vi "main.vi"() -> ()   [LabVIEW 2013]
uses:
  <vilib>/addons/internet/telnet/telnet.llb/Telnet Session.ctl
  <vilib>/Platform/TimedLoop/XDataNode/timing_clust.ctl
  <vilib>/Platform/TimedLoop/XDataNode/nitl_modes.ctl
  <vilib>/Platform/TimedLoop/XDataNode/wakeup.ctl
  FGV/STANDARD/Action.ctl
  <vilib>/Utility/config.llb/Read Key (Path).vi
  <vilib>/Utility/config.llb/Write Key (Path).vi
  <vilib>/Instr/_visa.llb/VISA Configure Serial Port (Instr).vi
  <vilib>/Platform/TimedLoop/XDataNode/XDataNode.xnode
  <vilib>/Platform/TimedLoop/XDataNode/XDNodeRunTimeDep.lvlib
  <vilib>/Utility/config.llb/NI_LVConfig.lvlib
panel:
  out "SettingsFile":path=path "D:/JD/PROJETS/wrk/WORKING_DIR"
  out "Tftp":T1={"HostIP"="192.168.1.200", "HostPort"=23, "ClientIP"="192.168.1.200"}
  out "Telnet":cluster{"HostIP":string, "HostPort":u16}={"HostIP"="192.168.1.200", "HostPort"=23}
  out "Error Out":errorcluster caption="Sortie d'erreur"
  in  "Serial_Port":refnum<visa-resource-name> caption="Serial Port"
  out "Serial_Connected":bool caption="Serial"
  in  "Serial_Connect":bool caption="Cmd_Tx"
  in  "Serial_Clear":bool
  in  "Serial_Console":string caption="Console"
  out "telnet connection":T2
  in  "BTN_Quit":bool
  in  "LauncherRef":refnum<vi>
  in  "entrée d'erreur":errorcluster caption="sortie d'erreur"
  out "sortie d'erreur":errorcluster
  in  "ONGLETS":enum32{"CONFIGURATION", "LOW_LEVEL", "COMMANDS"}(tab)
  in  "Host_IpAddress":string="192.168.1.200" caption="GHB Address"
  in  "MyIpList":string(combo) caption="My IP address"
  in  "WorkingDir":path=path "D:/JD/PROJETS/wrk/WORKING_DIR"
  in  "Host_TelnetPort":u16=23 caption="Telnet Port"
  in  "Host_TftpPort":u16=69 caption="Tftp Port"
  in  "OpenWorkingDir":bool
  in  "Telnet_Connect":bool
  in  "Telnet_Tx":bool caption="Cmd_Tx"
  in  "Telnet_Cmd":string caption="Cmd"
  in  "Telnet_Console":string caption="Console"
  in  "Telnet_Clear":bool
  out "Telnet_Connected":bool caption="Telnet"
  in  "Tftp_RemotePath":string
  out "Tftp_Status":bool caption="Status"
  in  "Tftp_LocalPath":path=path "D:/JD/PROJETS/wrk/TESTS"
  in  "Tftp_Get":bool
  in  "Tftp_Put":bool
  out "Tftp_Connected":bool caption="Tftp"
  in  "Cmd_ReservoirSet":bool caption="Cmd_Tx"
  in  "Cmd_ReservoirGet":bool caption="Cmd_Tx"
  in  "Cmd_Arroser":bool caption="Cmd_Tx"
  in  "Cmd_GetState":bool caption="Cmd_Tx"
  in  "Cmd_PutFile":bool caption="Cmd_Tx"
  in  "Cmd_GetFile":bool caption="Cmd_Tx"
  in  "FileList":i32(listbox)
  in  "Cmd_Reboot":bool caption="Cmd_Tx"
  in  "Cmd_ListFiles":bool caption="Cmd_Tx"
  in  "Cmd_Rename":bool caption="Cmd_Tx"
  in  "Cmd_Delete":bool caption="Cmd_Tx"
  in  "Cmd_Parameters":string caption="Parameters"
  in  "Cmd_Read":bool caption="Cmd_Tx"
  in  "Cmd_RtcGet":bool caption="Cmd_Tx"
  in  "Cmd_RtcSet":bool caption="Cmd_Tx"
  in  "Cmd_LogsGet":bool caption="Cmd_Tx"
  in  "Cmd_LogsClear":bool caption="Cmd_Tx"
  in  "Cmd_Console":string caption="Console"
  in  "Cmd_Clear":bool
  # "SERIAL"
  # "CONFIGURATION"
  # "TELNET"
  # "TFTP"
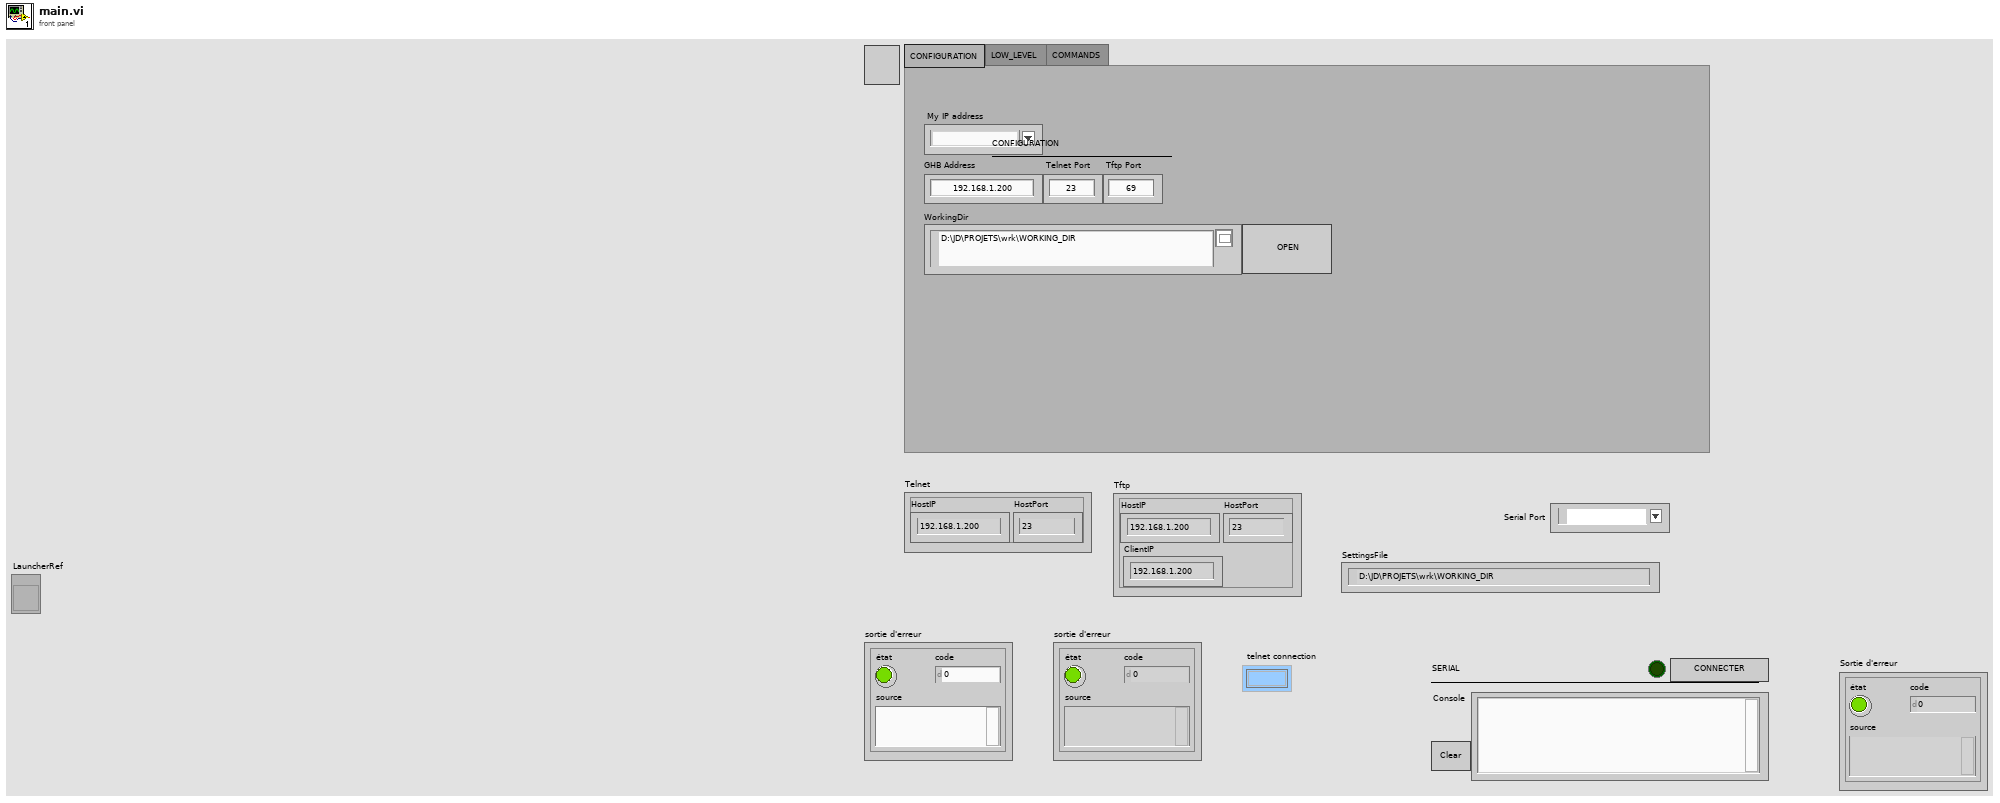
[diagram p1: front panel]
types:
  T1 = cluster{"HostIP":string, "HostPort":u16, "ClientIP":string}
  T2 = typedef "Telnet Session.ctl" = refnum<k1>
  T3 = enum32{"invalid app kind", "Development System", "Run Time System", "Student Edition", "Embedded LabVIEW", "Evaluation", "Custom"}
  T4 = typedef "Action.ctl" = enum16{"SET", "GET"}
  T5 = typedef "CtrlRef.ctl" = cluster{"Name":string, "Ref":refnum<vi>, "ClassName":string}
  T6 = typedef "NI_LVConfig.lvlib/Config Data RefNum.ctl" = refnum<k1>
  T7 = typedef "XDNodeRunTimeDep.lvlib/timing_clust.ctl" = cluster{"Expected End [f-1]":u64, "Actual End [f-1]":u64, "Finished Late? [f-1]":bool, "Expected End [i-1]":u64, "Actual End [i-1]":u64, "Finished Late? [i-1]":bool, "Expected Start [i]":u64, "Actual Start [i]":u64, "Expected Start [f]":u64, "Actual Start [f]":u64, "Source Name":string, "Structure Name":string, "Period":i64, "Deadline":i64, "Offset":i64, "Start":i64, "Priority":i32, "Timeout":i32, "Mode":T8, "Wakeup Reason":T9, "Error":errorcluster, "Source Type":string, "Secondary Source Type":string, "Global End Time":u64, "Global Start Time":u64, "Frame Duration":u64, "Iteration Duration":u64, "Assigned CPU":i32, "I/O Scan Engine Mode":u32}
  T8 = typedef "XDNodeRunTimeDep.lvlib/nitl_modes.ctl" = enum32{"No Change", "Process missed periods, maintain original phase", "Discard missed periods, maintain original phase", "Process missed periods, ignore original phase", "Discard missed periods, ignore original phase"}
  T9 = typedef "XDNodeRunTimeDep.lvlib/wakeup.ctl" = enum32{"Normal", "Aborted", "Asynchronous wakeup", "Timing source error", "Timed loop error", "Timeout"}
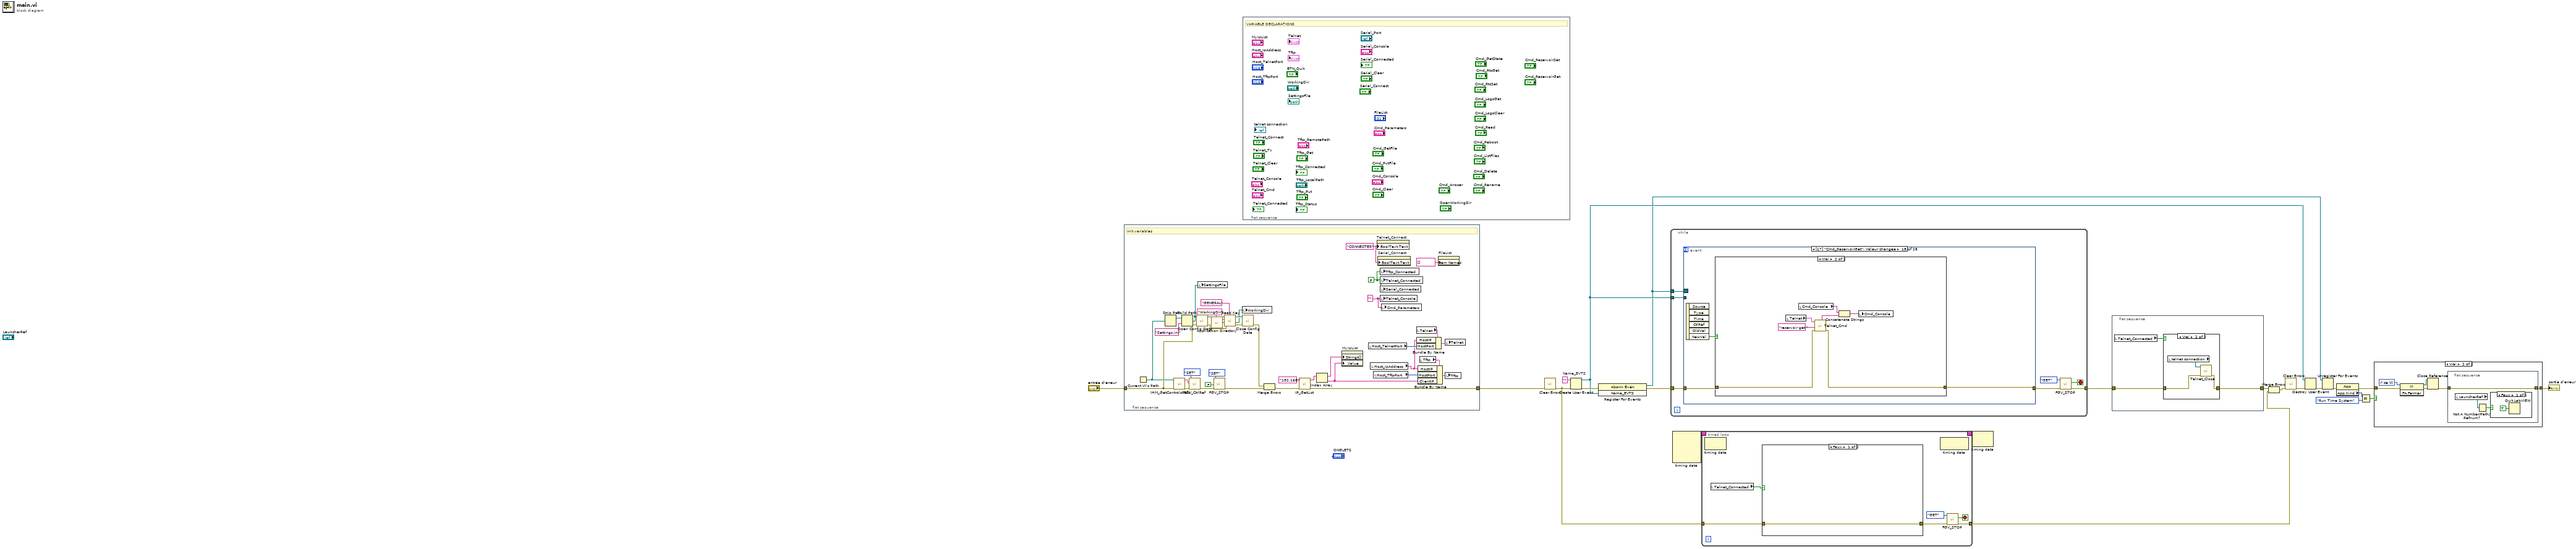
[diagram p0: block diagram]
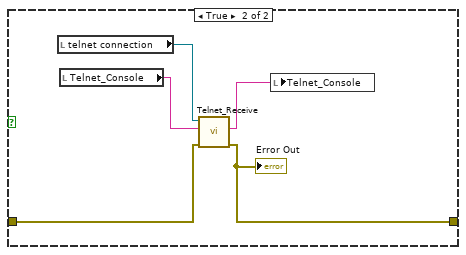
[diagram p3: hidden frame]
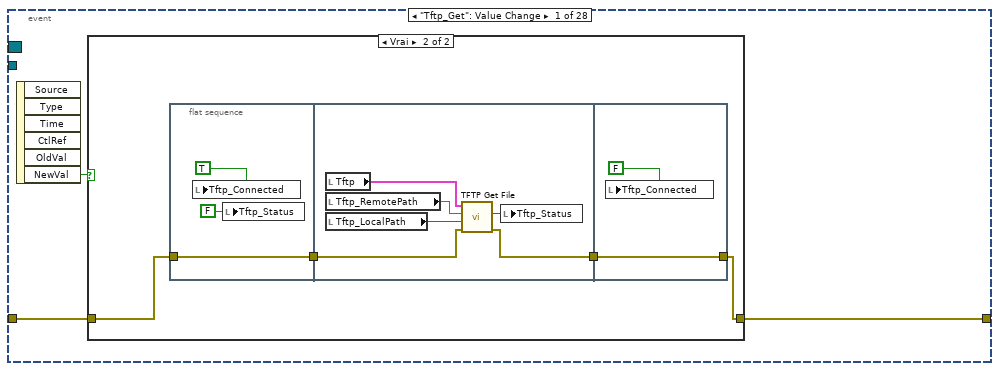
[diagram p6: hidden frame]
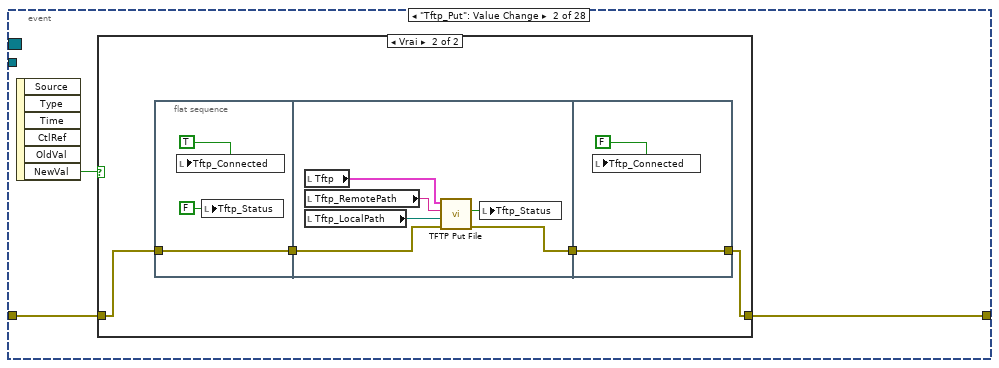
[diagram p8: hidden frame]
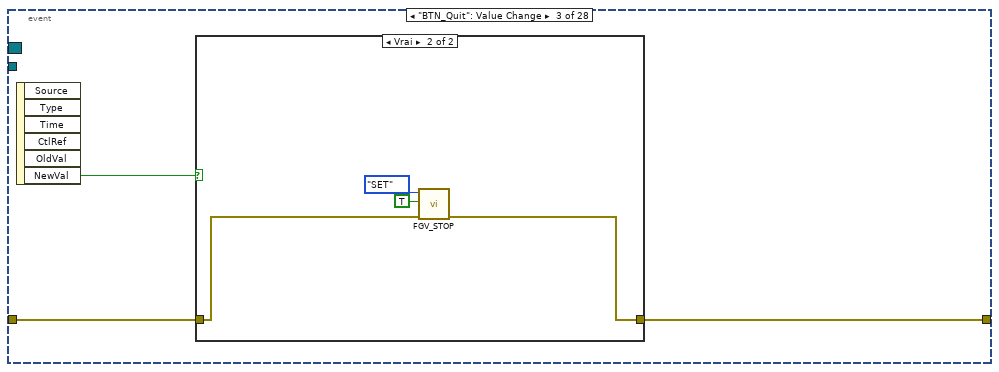
[diagram p10: hidden frame]
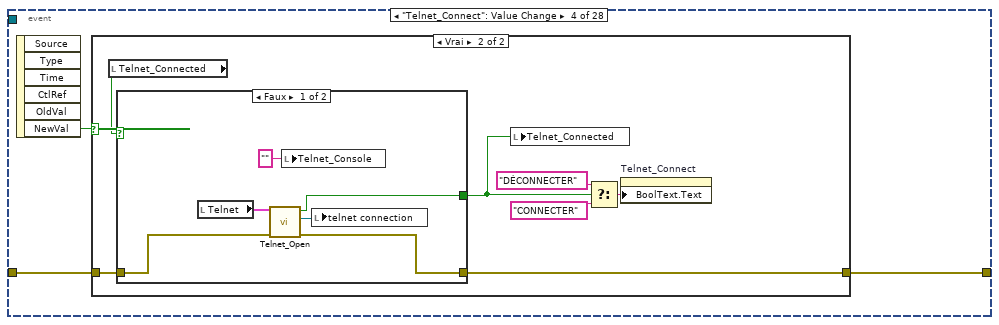
[diagram p12: hidden frame]
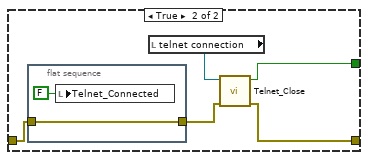
[diagram p14: hidden frame]
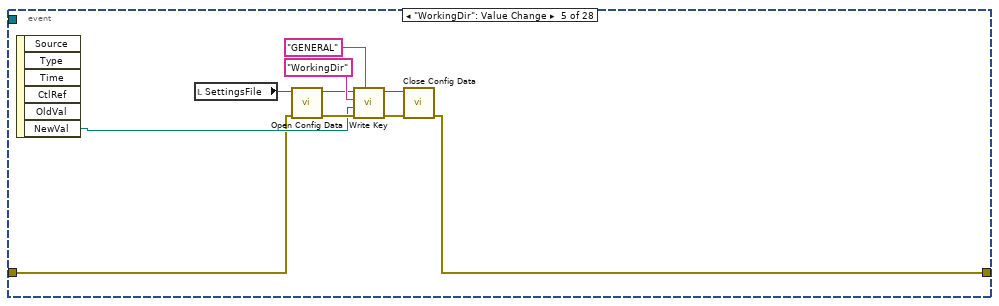
[diagram p15: hidden frame]
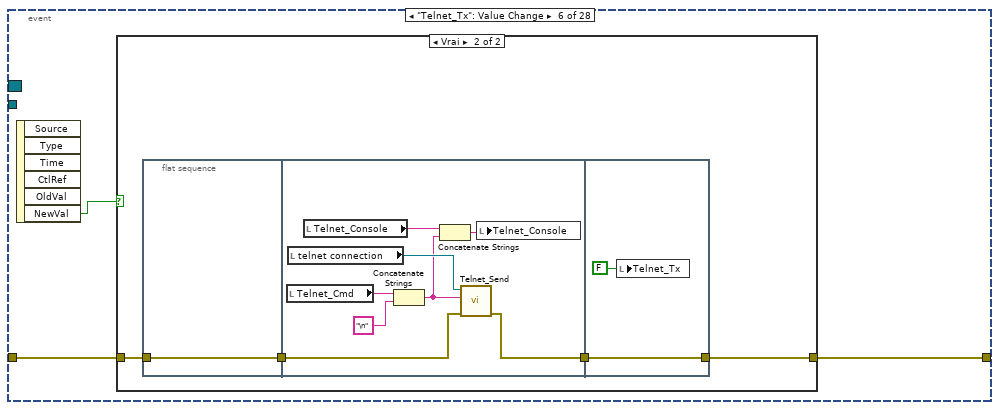
[diagram p16: hidden frame]
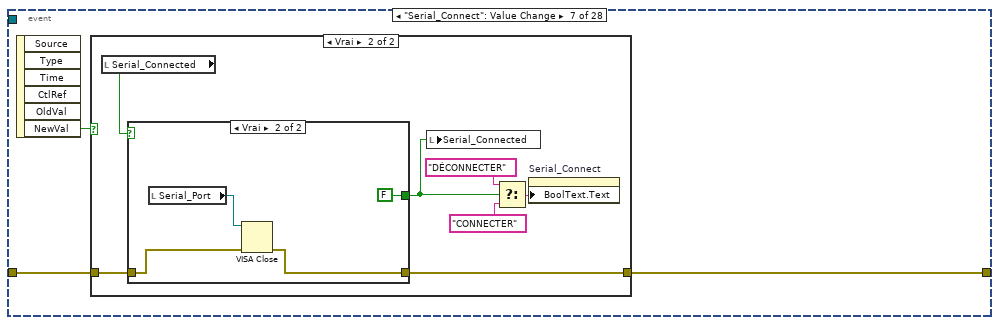
[diagram p18: hidden frame]
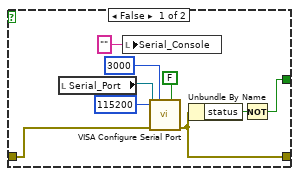
[diagram p20: hidden frame]
diagram:
  w22 = ""  # Name_EVTS
  n1 = flat-sequence {
    tunnel: [w51] -> w19
    tunnel: "entrée d'erreur" -> [w25]
    frame #0 {
      w54 = "" ("Telnet_Console")
      w56 = FALSE ("Telnet_Connected")
      w57 = "CONNECTER" ("Texte booléen.Texte")
      # "Init variables"
      n2 = Current VI's Path() -> (path=w37:path)
      n3 = Strip Path(path=w37) -> (stripped path=w38:path)  [unwired: 1 out]
      n4 = call "IHM_GetControlsRefs.vi"("Error In"=w25, "chemin du VI"=w37) -> ("Error Out"=w50:errorcluster, "CtrlsRefs_OUT"=w48:T5[])  [unwired: 8 in]
      n5 = Build Path(base path=w38, name or relative path="Settings.ini" ("nom ou chemin relatif")) -> (appended path=w24:path)
      n6 = call "FGV_CtrlRef.vi"("error in (no error)"=w50, "CtrlsRefs_IN"=w48, "Action"=Action."SET") -> ("error out"=w47:errorcluster)  [unwired: 7 in, 1 out]
      n7 = call <vilib>:"Open Config Data.vi"("error in (no error)"=w25, "configuration file path"=w24) -> ("error out"=w26:errorcluster, "refnum"=w35:T6)  [unwired: 7 in, 1 out]
      n8 = local write "SettingsFile"(w24) -> ()
      n9 = call <vilib>:"Application Directory.vi"() -> ("Application Directory"=w32:path)
      n10 = call "FGV_STOP.vi"("error in (no error)"=w47, "Data_IN"=FALSE, "Action"=Action."SET") -> ("error out"=w29:errorcluster)  [unwired: 7 in, 1 out]
      n11 = call-poly <vilib>:"Read Key.vi"("section"="GENERAL", "error in (no error)"=w26, "default value"=w32, "key"="WorkingDir", "refnum"=w35) -> ("error out"=w27:errorcluster, "value"=w31:path, "refnum out"=w34:T6)  [unwired: 3 in, 1 out]
      n12 = local write "WorkingDir"(w31) -> ()
      n13 = call <vilib>:"Close Config Data.vi"("error in (no error)"=w27, "refnum"=w34) -> ("error out"=w28:errorcluster)  [unwired: 8 in, 1 out]
      n14 = Merge Errors(w28, w29) -> (w30:errorcluster)
      n15 = call "IP_GetList.vi"("Error In"=w30, "MustContain"="192.168." ("expression régulière")) -> ("Error Out"=w51:errorcluster, "IP_List"=w52:string[])  [unwired: 8 in]
      n16 = Index Array(array=w52) -> (element=w42:string)  [unwired: 1 in]
      n17 = property on="MyIpList" class="ChneDér"("Strings[]"=w52, "Value"=w42) -> ()  [unwired: 2 in, 2 out]
      n18 = local read "Host_TelnetPort"() -> (w40:u16)
      n19 = local read "Host_IpAddress"() -> (w39:string)
      n20 = local read "Host_TftpPort"() -> (w41:u16)
      n21 = property on="Telnet_Connect" class="Bool (strict)"("BoolText.Text"=w57) -> ()  [unwired: 2 in, 2 out]
      n22 = property on="Serial_Connect" class="Bool (strict)"("BoolText.Text"=w57) -> ()  [unwired: 2 in, 2 out]
      n23 = local write "Tftp_Connected"(w56) -> ()
      n24 = local write "Telnet_Connected"(w56) -> ()
      n25 = local write "Serial_Connected"(w56) -> ()
      n26 = local write "Telnet_Console"(w54) -> ()
      n27 = local write "Cmd_Parameters"(w54) -> ()
      n28 = local read "Telnet"() -> (w43:cluster{"HostIP":string, "HostPort":u16})
      n29 = Bundle By Name(cluster=w43, "HostIP"=w39, "HostPort"=w40) -> (w44:cluster{"HostIP":string, "HostPort":u16})
      n30 = local read "Tftp"() -> (w46:T1)
      n31 = Bundle By Name(cluster=w46, "HostIP"=w39, "HostPort"=w41, "ClientIP"=w42) -> (w45:T1)
      n32 = property on="FileList" class="LstDér (strict)"("Item Names"=string[] [] ("Noms d'éléments")) -> ()  [unwired: 2 in, 2 out]
      n33 = local write "Tftp"(w45) -> ()
      n34 = local write "Telnet"(w44) -> ()
    }
  }
  n35 = flat-sequence {
    frame #0 {
      # "VARIABLE DECLARATIONS"
    }
  }
  n36 = call <vilib>:"Clear Errors.vi"("error in (no error)"=w19) -> ("error out"=w4:errorcluster)  [unwired: 6 in]
  n37 = Create User Event(user event datatype=w22, error in=w4) -> (user event=w9:refnum<user-event>, error out=w21:errorcluster)
  n38 = register-events(error in=w21, w9) -> (reference out=w8:refnum<event-registration>, error out=w7:errorcluster)  [unwired: 1 in]
  n39 = while {
    tunnel: w9 -> [w65]
    tunnel: w8 -> [w64]
    tunnel: [w62] -> w2
    tunnel: w7 -> [w60]
    stop <- w63 stop-if-true
    n40 = event shown="[17] \"Cmd_ReservoirGet\": Valeur changée" {
      selector: w64 -> [_ _ _ _ _ _ _ _ _ _ _ _ _ _ _ _ _ _ _ _ _ _ _ _ _ _ _ _]
      dyn-events: _ -> [_ _ _ _ _ _ _ _ _ _ _ _ _ _ _ _ _ _ _ _ _ _ _ _ _ _ _ _]
      timeout: _ -> [_ _ _ _ _ _ _ _ _ _ _ _ _ _ _ _ _ _ _ _ _ _ _ _ _ _ _ _]
      tunnel: w65 -> [_ _ _ _ _ _ _ _ _ _ _ _ _ _ _ _ _ _ _ _ _ _ _ _ _ _ _ _]
      tunnel: [w69 w87 w106 w115 w139 w149 w167 w192 w203 w214 w227 w239 w245 w248 w251 w254 w267 w280 w291 w304 w315 w329 w366 w372 w376 w380 w382 w394] -> w61
      tunnel: w60 -> [w68 w88 w105 w114 w140 w148 w168 w191 w204 w215 w228 w240 w245 w248 w251 w255 w268 w281 w292 w305 w316 w328 w366 w372 w376 w380 w383 w395]
      event "Tftp_Get": Value Change {
        n41 = event-data() -> ("NewVal"=w67:bool)  [unwired: 1 in, 5 out]
        n42 = case shown="Vrai" w67 {
          tunnel: [w70 w72] -> w69
          tunnel: w68 -> [w70 w73]
          frame False {
          }
          frame True {
            n43 = flat-sequence {
              tunnel: [w76] -> w74
              tunnel: w73 -> [w76]
              tunnel: w74 -> [w79]
              tunnel: [w78] -> w71
              tunnel: [w85] -> w72
              tunnel: w71 -> [w85]
              frame #0 {
                n44 = local write "Tftp_Connected"(TRUE ("Tftp_Connected")) -> ()
                n45 = local write "Tftp_Status"(FALSE ("TFTP_Status")) -> ()
              }
              frame #1 {
                n46 = local read "Tftp"() -> (w82:T1)
                n47 = local read "Tftp_RemotePath"() -> (w81:string)
                n48 = local read "Tftp_LocalPath"() -> (w80:path)
                n49 = call "TFTP Get File.vi"("error in (no error)"=w79, "local path"=w80, "remote path"=w81, "IpConf"=w82) -> ("error out"=w78:errorcluster, "Status"=w83:bool)  [unwired: 5 in, 1 out]
                n50 = local write "Tftp_Status"(w83) -> ()
              }
              frame #2 {
                n51 = local write "Tftp_Connected"(FALSE ("Tftp_Connected")) -> ()
              }
            }
          }
        }
      }
      event "Tftp_Put": Value Change {
        n52 = event-data() -> ("NewVal"=w86:bool)  [unwired: 1 in, 5 out]
        n53 = case shown="Vrai" w86 {
          tunnel: [w89 w91] -> w87
          tunnel: w88 -> [w89 w93]
          frame False {
          }
          frame True {
            n54 = flat-sequence {
              tunnel: w93 -> [w95]
              tunnel: [w95] -> w92
              tunnel: w92 -> [w98]
              tunnel: [w97] -> w90
              tunnel: [w104] -> w91
              tunnel: w90 -> [w104]
              frame #0 {
                n55 = local write "Tftp_Connected"(TRUE ("Tftp_Connected")) -> ()
                n56 = local write "Tftp_Status"(FALSE ("TFTP_Status")) -> ()
              }
              frame #1 {
                n57 = local read "Tftp"() -> (w101:T1)
                n58 = local read "Tftp_RemotePath"() -> (w100:string)
                n59 = local read "Tftp_LocalPath"() -> (w99:path)
                n60 = call "TFTP Put File.vi"("error in (no error)"=w98, "local path"=w99, "remote path"=w100, "IpConf"=w101) -> ("error out"=w97:errorcluster, "Status"=w102:bool)  [unwired: 5 in, 1 out]
                n61 = local write "Tftp_Status"(w102) -> ()
              }
              frame #2 {
                n62 = local write "Tftp_Connected"(FALSE ("Tftp_Connected")) -> ()
              }
            }
          }
        }
      }
      event "BTN_Quit": Value Change {
        n63 = event-data() -> ("NewVal"=w107:bool)  [unwired: 1 in, 5 out]
        n64 = case shown="Vrai" w107 {
          tunnel: [w108 w110] -> w106
          tunnel: w105 -> [w108 w111]
          frame False {
          }
          frame True {
            n65 = call "FGV_STOP.vi"("error in (no error)"=w111, "Data_IN"=TRUE, "Action"=Action."SET") -> ("error out"=w110:errorcluster)  [unwired: 7 in, 1 out]
          }
        }
      }
      event "Telnet_Connect": Value Change {
        n66 = event-data() -> ("NewVal"=w113:bool)  [unwired: 1 in, 5 out]
        n67 = case shown="Vrai" w113 {
          tunnel: [w116 w122] -> w115
          tunnel: w114 -> [w116 w123]
          frame False {
          }
          frame True {
            n68 = local read "Telnet_Connected"() -> (w121:bool)
            n69 = case shown="Faux" w121 {
              tunnel: w123 -> [w129 w130]
              tunnel: [w127 w134] -> w122
              tunnel: [w126 w132] -> w117
              frame False {
                n70 = local read "Telnet"() -> (w124:cluster{"HostIP":string, "HostPort":u16})
                n71 = call "Telnet_Open.vi"("Error In"=w129, "Telnet"=w124) -> ("Error Out"=w127:errorcluster, "telnet connection"=w128:T2, "Status"=w126:bool)  [unwired: 7 in]
                n72 = local write "Telnet_Console"("" ("Telnet_Console")) -> ()
                n73 = local write "telnet connection"(w128) -> ()
              }
              frame True {
                n74 = flat-sequence {
                  tunnel: [w136] -> w131
                  tunnel: w130 -> [w136]
                  frame #0 {
                    n75 = local write "Telnet_Connected"(FALSE ("Telnet_Connected")) -> ()
                  }
                }
                n76 = local read "telnet connection"() -> (w133:T2)
                n77 = call "Telnet_Close.vi"("Error In"=w131, "telnet connection"=w133) -> ("Error Out"=w134:errorcluster, "Connecté"=w132:bool)  [unwired: 8 in]
              }
            }
            n78 = local write "Telnet_Connected"(w117) -> ()
            n79 = Select(t="DÉCONNECTER" ("Texte booléen.Texte"), s=w117, f="CONNECTER" ("Texte booléen.Texte")) -> (s? t:f=w118:string)
            n80 = property on="Telnet_Connect" class="Bool (strict)"("BoolText.Text"=w118) -> ()  [unwired: 2 in, 2 out]
          }
        }
      }
      event "WorkingDir": Value Change {
        n81 = event-data() -> ("NewVal"=w141:path)  [unwired: 1 in, 5 out]
        n82 = local read "SettingsFile"() -> (w138:path)
        n83 = call <vilib>:"Open Config Data.vi"("error in (no error)"=w140, "configuration file path"=w138) -> ("error out"=w146:errorcluster, "refnum"=w142:T6)  [unwired: 7 in, 1 out]
        n84 = call-poly <vilib>:"Write Key.vi"("section"="GENERAL", "error in (no error)"=w146, "value"=w141, "key"="WorkingDir", "refnum"=w142) -> ("error out"=w145:errorcluster, "refnum out"=w143:T6)  [unwired: 4 in, 1 out]
        n85 = call <vilib>:"Close Config Data.vi"("error in (no error)"=w145, "refnum"=w143) -> ("error out"=w139:errorcluster)  [unwired: 8 in, 1 out]
      }
      event "Telnet_Tx": Value Change {
        n86 = event-data() -> ("NewVal"=w147:bool)  [unwired: 1 in, 5 out]
        n87 = case shown="Vrai" w147 {
          tunnel: [w150 w153] -> w149
          tunnel: w148 -> [w150 w154]
          frame False {
          }
          frame True {
            n88 = flat-sequence {
              tunnel: w154 -> [w155]
              tunnel: [w155] -> w152
              tunnel: w152 -> [w162]
              tunnel: [w161] -> w151
              tunnel: [w165] -> w153
              tunnel: w151 -> [w165]
              frame #0 {
              }
              frame #1 {
                n89 = local read "Telnet_Cmd"() -> (w158:string)
                n90 = local read "telnet connection"() -> (w163:T2)
                n91 = local read "Telnet_Console"() -> (w160:string)
                n92 = Concatenate Strings(w158, "\n") -> (w156:string)
                n93 = Concatenate Strings(w160, w156) -> (w159:string)
                n94 = call "Telnet_Send.vi"("Error In"=w162, "Data in"=w156, "telnet connection in"=w163) -> ("Error Out"=w161:errorcluster)  [unwired: 7 in, 1 out]
                n95 = local write "Telnet_Console"(w159) -> ()
              }
              frame #2 {
                n96 = local write "Telnet_Tx"(FALSE ("Telnet_Tx")) -> ()
              }
            }
          }
        }
      }
      event "Serial_Connect": Value Change {
        n97 = event-data() -> ("NewVal"=w166:bool)  [unwired: 1 in, 5 out]
        n98 = case shown="Vrai" w166 {
          tunnel: [w169 w175] -> w167
          tunnel: w168 -> [w169 w176]
          frame False {
          }
          frame True {
            n99 = local read "Serial_Connected"() -> (w171:bool)
            n100 = case shown="Vrai" w171 {
              tunnel: w176 -> [w182 w188]
              tunnel: [w179 w187] -> w175
              tunnel: [w177 FALSE] -> w172
              frame False {
                n101 = local read "Serial_Port"() -> (w183:refnum<visa-resource-name>)
                n102 = local write "Serial_Console"("" ("Telnet_Console")) -> ()
                n103 = call-poly "VISA Configure Serial Port"("VISA resource name"=w183, "timeout (10sec)"=u32 3000, "Enable Termination\nChar (T)"=FALSE ("Enable Termination\nChar (T)"), "baud rate (9600)"=u32 115200, "error in (no error)"=w182) -> ("error out"=w179:errorcluster)  [unwired: 9 in, 1 out]
                n104 = Unbundle By Name(w179) -> ("status"=w178:bool)
                n105 = Not(x=w178) -> (.not. x?=w177:bool)
              }
              frame True {
                n106 = local read "Serial_Port"() -> (w189:refnum<visa-resource-name>)
                n107 = VISA Close(VISA resource name=w189, error in (no error)=w188) -> (error out=w187:errorcluster)
              }
            }
            n108 = local write "Serial_Connected"(w172) -> ()
            n109 = Select(t="DÉCONNECTER" ("Texte booléen.Texte"), s=w172, f="CONNECTER" ("Texte booléen.Texte")) -> (s? t:f=w170:string)
            n110 = property on="Serial_Connect" class="Bool (strict)"("BoolText.Text"=w170) -> ()  [unwired: 2 in, 2 out]
          }
        }
      }
      event "Cmd_ListFiles": Value Change {
        n111 = event-data() -> ("NewVal"=w190:bool)  [unwired: 1 in, 5 out]
        n112 = case shown="Vrai" w190 {
          tunnel: [w193 w198] -> w192
          tunnel: w191 -> [w193 w200]
          frame False {
          }
          frame True {
            n113 = local read "Telnet"() -> (w201:cluster{"HostIP":string, "HostPort":u16})
            n114 = local read "Cmd_Console"() -> (w196:string)
            n115 = call "Telnet_Cmd.vi"("Error In"=w200, "Cmd"="ls", "Host"=w201) -> ("Error Out"=w198:errorcluster, "DataLines"=w197:string[], "Console"=w194:string)  [unwired: 5 in, 1 out]
            n116 = property on="FileList" class="LstDér (strict)"("Item Names"=w197) -> ()  [unwired: 2 in, 2 out]
            n117 = Concatenate Strings(w196, w194) -> (w195:string)
            n118 = local write "Cmd_Console"(w195) -> ()
          }
        }
      }
      event "Cmd_Reboot": Value Change {
        n119 = event-data() -> ("NewVal"=w202:bool)  [unwired: 1 in, 5 out]
        n120 = case shown="Vrai" w202 {
          tunnel: [w205 w209] -> w203
          tunnel: w204 -> [w205 w211]
          frame False {
          }
          frame True {
            n121 = local read "Telnet"() -> (w212:cluster{"HostIP":string, "HostPort":u16})
            n122 = local read "Cmd_Console"() -> (w208:string)
            n123 = call "Telnet_Cmd.vi"("Error In"=w211, "Cmd"="reboot", "Host"=w212) -> ("Error Out"=w209:errorcluster, "Console"=w206:string)  [unwired: 5 in, 2 out]
            n124 = Concatenate Strings(w208, w206) -> (w207:string)
            n125 = local write "Cmd_Console"(w207) -> ()
          }
        }
      }
      event "Cmd_Rename": Value Change {
        n126 = event-data() -> ("NewVal"=w213:bool)  [unwired: 1 in, 5 out]
        n127 = case shown="Vrai" w213 {
          tunnel: [w216 w223] -> w214
          tunnel: w215 -> [w216 w224]
          frame False {
          }
          frame True {
            n128 = local read "Cmd_Parameters"() -> (w220:string)
            n129 = local read "Telnet"() -> (w225:cluster{"HostIP":string, "HostPort":u16})
            n130 = Concatenate Strings("rename " ("Cmd"), w220) -> (w221:string)
            n131 = local read "Cmd_Console"() -> (w218:string)
            n132 = call "Telnet_Cmd.vi"("Error In"=w224, "Cmd"=w221, "Host"=w225) -> ("Error Out"=w223:errorcluster, "Console"=w219:string)  [unwired: 5 in, 2 out]
            n133 = Concatenate Strings(w218, w219) -> (w217:string)
            n134 = local write "Cmd_Console"(w217) -> ()
          }
        }
      }
      event "Cmd_Delete": Value Change {
        n135 = event-data() -> ("NewVal"=w226:bool)  [unwired: 1 in, 5 out]
        n136 = case shown="Vrai" w226 {
          tunnel: [w229 w236] -> w227
          tunnel: w228 -> [w229 w237]
          frame False {
          }
          frame True {
            n137 = local read "Cmd_Parameters"() -> (w233:string)
            n138 = local read "Telnet"() -> (w238:cluster{"HostIP":string, "HostPort":u16})
            n139 = Concatenate Strings("delete " ("Cmd"), w233) -> (w234:string)
            n140 = local read "Cmd_Console"() -> (w232:string)
            n141 = call "Telnet_Cmd.vi"("Error In"=w237, "Cmd"=w234, "Host"=w238) -> ("Error Out"=w236:errorcluster, "Console"=w230:string)  [unwired: 5 in, 2 out]
            n142 = Concatenate Strings(w232, w230) -> (w231:string)
            n143 = local write "Cmd_Console"(w231) -> ()
          }
        }
      }
      event "FileList": Double Click {
        n144 = event-data() -> ("Row"=w242:i32)  [unwired: 1 in, 8 out]
        n145 = property on="FileList" class="LstDér (strict)"(error in=w240) -> (error out=w239:errorcluster, "Item Names"=w243:string[])  [unwired: 1 in, 1 out]
        n146 = Index Array(array=w243, index=w242) -> (element=w241:string)
        n147 = local write "Cmd_Parameters"(w241) -> ()
      }
      event "Telnet_Clear": Value Change {
        n148 = event-data() -> ("NewVal"=w244:bool)  [unwired: 1 in, 5 out]
        n149 = case shown="Vrai" w244 {
          frame False {
          }
          frame True {
            n150 = local write "Telnet_Console"("" ("Console")) -> ()
          }
        }
      }
      event "Cmd_Clear": Value Change {
        n151 = event-data() -> ("NewVal"=w247:bool)  [unwired: 1 in, 5 out]
        n152 = case shown="Vrai" w247 {
          frame False {
          }
          frame True {
            n153 = local write "Cmd_Console"("" ("Console")) -> ()
          }
        }
      }
      event "OpenWorkingDir": Value Change {
        n154 = event-data() -> ("NewVal"=w250:bool)  [unwired: 1 in, 5 out]
        n155 = case shown="Vrai" w250 {
          frame False {
          }
          frame True {
            n156 = local read "WorkingDir"() -> (w252:path)
            n157 = call "CmdStart.vi"("Path"=w252) -> ()  [unwired: 6 in, 1 out]
          }
        }
      }
      event "Cmd_Read": Value Change {
        n158 = event-data() -> ("NewVal"=w253:bool)  [unwired: 1 in, 5 out]
        n159 = case shown="Vrai" w253 {
          tunnel: [w256 w263] -> w254
          tunnel: w255 -> [w256 w264]
          frame False {
          }
          frame True {
            n160 = local read "Cmd_Parameters"() -> (w260:string)
            n161 = local read "Telnet"() -> (w265:cluster{"HostIP":string, "HostPort":u16})
            n162 = Concatenate Strings("read " ("Cmd"), w260) -> (w261:string)
            n163 = local read "Cmd_Console"() -> (w258:string)
            n164 = call "Telnet_Cmd.vi"("Error In"=w264, "Cmd"=w261, "Host"=w265) -> ("Error Out"=w263:errorcluster, "Console"=w259:string)  [unwired: 5 in, 2 out]
            n165 = Concatenate Strings(w258, w259) -> (w257:string)
            n166 = local write "Cmd_Console"(w257) -> ()
          }
        }
      }
      event "Cmd_Arroser": Value Change {
        n167 = event-data() -> ("NewVal"=w266:bool)  [unwired: 1 in, 5 out]
        n168 = case shown="Vrai" w266 {
          tunnel: [w269 w276] -> w267
          tunnel: w268 -> [w269 w277]
          frame False {
          }
          frame True {
            n169 = local read "Cmd_Parameters"() -> (w273:string)
            n170 = local read "Telnet"() -> (w278:cluster{"HostIP":string, "HostPort":u16})
            n171 = Concatenate Strings("arroser " ("Cmd"), w273) -> (w274:string)
            n172 = local read "Cmd_Console"() -> (w271:string)
            n173 = call "Telnet_Cmd.vi"("Error In"=w277, "Cmd"=w274, "Host"=w278) -> ("Error Out"=w276:errorcluster, "Console"=w272:string)  [unwired: 5 in, 2 out]
            n174 = Concatenate Strings(w271, w272) -> (w270:string)
            n175 = local write "Cmd_Console"(w270) -> ()
          }
        }
      }
      event "Cmd_ReservoirGet": Value Change {
        n176 = event-data() -> ("NewVal"=w279:bool)  [unwired: 1 in, 5 out]
        n177 = case shown="Vrai" w279 {
          tunnel: [w282 w287] -> w280
          tunnel: w281 -> [w282 w288]
          frame False {
          }
          frame True {
            n178 = local read "Telnet"() -> (w289:cluster{"HostIP":string, "HostPort":u16})
            n179 = local read "Cmd_Console"() -> (w285:string)
            n180 = call "Telnet_Cmd.vi"("Error In"=w288, "Cmd"="reservoir get ", "Host"=w289) -> ("Error Out"=w287:errorcluster, "Console"=w286:string)  [unwired: 5 in, 2 out]
            n181 = Concatenate Strings(w285, w286) -> (w284:string)
            n182 = local write "Cmd_Console"(w284) -> ()
          }
        }
      }
      event "Cmd_ReservoirSet": Value Change {
        n183 = event-data() -> ("NewVal"=w290:bool)  [unwired: 1 in, 5 out]
        n184 = case shown="Vrai" w290 {
          tunnel: [w293 w300] -> w291
          tunnel: w292 -> [w293 w301]
          frame False {
          }
          frame True {
            n185 = local read "Cmd_Parameters"() -> (w297:string)
            n186 = local read "Telnet"() -> (w302:cluster{"HostIP":string, "HostPort":u16})
            n187 = Concatenate Strings("reservoir set " ("Cmd"), w297) -> (w298:string)
            n188 = local read "Cmd_Console"() -> (w295:string)
            n189 = call "Telnet_Cmd.vi"("Error In"=w301, "Cmd"=w298, "Host"=w302) -> ("Error Out"=w300:errorcluster, "Console"=w296:string)  [unwired: 5 in, 2 out]
            n190 = Concatenate Strings(w295, w296) -> (w294:string)
            n191 = local write "Cmd_Console"(w294) -> ()
          }
        }
      }
      event "Cmd_RtcGet": Value Change {
        n192 = event-data() -> ("NewVal"=w303:bool)  [unwired: 1 in, 5 out]
        n193 = case shown="Vrai" w303 {
          tunnel: [w306 w311] -> w304
          tunnel: w305 -> [w306 w312]
          frame False {
          }
          frame True {
            n194 = local read "Telnet"() -> (w313:cluster{"HostIP":string, "HostPort":u16})
            n195 = local read "Cmd_Console"() -> (w309:string)
            n196 = call "Telnet_Cmd.vi"("Error In"=w312, "Cmd"="rtc get ", "Host"=w313) -> ("Error Out"=w311:errorcluster, "Console"=w310:string)  [unwired: 5 in, 2 out]
            n197 = Concatenate Strings(w309, w310) -> (w308:string)
            n198 = local write "Cmd_Console"(w308) -> ()
          }
        }
      }
      event "Cmd_RtcSet": Value Change {
        n199 = event-data() -> ("NewVal"=w314:bool)  [unwired: 1 in, 5 out]
        n200 = case shown="Vrai" w314 {
          tunnel: [w317 w324] -> w315
          tunnel: w316 -> [w317 w325]
          frame False {
          }
          frame True {
            n201 = local read "Cmd_Parameters"() -> (w321:string)
            n202 = local read "Telnet"() -> (w326:cluster{"HostIP":string, "HostPort":u16})
            n203 = Concatenate Strings("rtc set " ("Cmd"), w321) -> (w322:string)
            n204 = local read "Cmd_Console"() -> (w319:string)
            n205 = call "Telnet_Cmd.vi"("Error In"=w325, "Cmd"=w322, "Host"=w326) -> ("Error Out"=w324:errorcluster, "Console"=w320:string)  [unwired: 5 in, 2 out]
            n206 = Concatenate Strings(w319, w320) -> (w318:string)
            n207 = local write "Cmd_Console"(w318) -> ()
          }
        }
      }
      event "Cmd_LogsGet": Value Change {
        n208 = event-data() -> ("NewVal"=w327:bool)  [unwired: 1 in, 5 out]
        n209 = case shown="Vrai" w327 {
          tunnel: [w330 w334] -> w329
          tunnel: w328 -> [w330 w340]
          frame False {
          }
          frame True {
            n210 = local read "Telnet"() -> (w341:cluster{"HostIP":string, "HostPort":u16})
            n211 = local read "Cmd_Console"() -> (w339:string)
            n212 = Concatenate Strings("ls " ("Cmd"), "LOGS" ("Cmd")) -> (w332:string)
            n213 = call "Telnet_Cmd.vi"("Error In"=w340, "Cmd"=w332, "Host"=w341) -> ("Error Out"=w335:errorcluster, "DataLines"=w336:string[], "Console"=w337:string)  [unwired: 5 in, 1 out]
            n214 = Concatenate Strings(w339, w337) -> (w338:string)
            n215 = property on="FileList" class="LstDér (strict)"("Item Names"=w336) -> ()  [unwired: 2 in, 2 out]
            n216 = for {
              tunnel: w336 -> [w342] mode=indexing
              tunnel: w335 -> [w347]
              tunnel: [w346] -> w334
              n217 = flat-sequence {
                tunnel: [w350] -> w345
                tunnel: w347 -> [w350]
                tunnel: [w348] -> w344
                tunnel: w342 -> [w348]
                tunnel: w345 -> [w355]
                tunnel: [w358] -> w343
                tunnel: w344 -> [w353]
                tunnel: [w362] -> w346
                tunnel: w343 -> [w362]
                frame #0 {
                  n218 = local write "Tftp_Connected"(TRUE ("Tftp_Connected")) -> ()
                  n219 = local write "Tftp_Status"(FALSE ("TFTP_Status")) -> ()
                }
                frame #1 {
                  n220 = Match Pattern(string=w353, regular expression="/" ("chaîne recherchée")) -> (after substring=w352:string)  [unwired: 1 in, 3 out]
                  n221 = local read "WorkingDir"() -> (w357:path)
                  n222 = Build Path(base path=w357, name or relative path=w352) -> (appended path=w356:path)
                  n223 = local read "Tftp"() -> (w359:T1)
                  n224 = call "TFTP Get File.vi"("error in (no error)"=w355, "local path"=w356, "remote path"=w353, "IpConf"=w359) -> ("error out"=w358:errorcluster, "Status"=w360:bool)  [unwired: 5 in, 1 out]
                  n225 = local write "Tftp_Status"(w360) -> ()
                }
                frame #2 {
                  n226 = local write "Tftp_Connected"(FALSE ("Tftp_Connected")) -> ()
                }
              }
            }
            n227 = local write "Cmd_Console"(w338) -> ()
          }
        }
      }
      event "MyIpList": Value Change {
        n228 = event-data() -> ("NewVal"=w364:string)  [unwired: 1 in, 5 out]
        n229 = local read "Tftp"() -> (w365:T1)
        n230 = Bundle By Name(cluster=w365, "ClientIP"=w364) -> (w363:T1)
        n231 = local write "Tftp"(w363) -> ()
      }
      event "Host_IpAddress": Value Change {
        n232 = event-data() -> ("NewVal"=w367:string)  [unwired: 1 in, 5 out]
        n233 = local read "Telnet"() -> (w368:cluster{"HostIP":string, "HostPort":u16})
        n234 = local read "Tftp"() -> (w371:T1)
        n235 = Bundle By Name(cluster=w371, "HostIP"=w367) -> (w370:T1)
        n236 = Bundle By Name(cluster=w368, "HostIP"=w367) -> (w369:cluster{"HostIP":string, "HostPort":u16})
        n237 = local write "Telnet"(w369) -> ()
        n238 = local write "Tftp"(w370) -> ()
      }
      event "Host_TelnetPort": Value Change {
        n239 = event-data() -> ("NewVal"=w373:u16)  [unwired: 1 in, 5 out]
        n240 = local read "Telnet"() -> (w374:cluster{"HostIP":string, "HostPort":u16})
        n241 = Bundle By Name(cluster=w374, "HostPort"=w373) -> (w375:cluster{"HostIP":string, "HostPort":u16})
        n242 = local write "Telnet"(w375) -> ()
      }
      event "Host_TftpPort": Value Change {
        n243 = event-data() -> ("NewVal"=w377:u16)  [unwired: 1 in, 5 out]
        n244 = local read "Tftp"() -> (w378:T1)
        n245 = Bundle By Name(cluster=w378, "HostPort"=w377) -> (w379:T1)
        n246 = local write "Tftp"(w379) -> ()
      }
      event "Cmd_GetFile": Value Change {
        n247 = event-data() -> ("NewVal"=w381:bool)  [unwired: 1 in, 5 out]
        n248 = case shown="Vrai" w381 {
          tunnel: [w384 w388] -> w382
          tunnel: w383 -> [w384 w391]
          frame False {
          }
          frame True {
            n249 = local read "Cmd_Parameters"() -> (w386:string)
            n250 = local read "WorkingDir"() -> (w390:path)
            n251 = String Subset(string=w386, offset (0)=1) -> (substring=w385:string)  [unwired: 1 in]
            n252 = Build Path(base path=w390, name or relative path=w385) -> (appended path=w389:path)
            n253 = local read "Tftp"() -> (w392:T1)
            n254 = call "TFTP Get File.vi"("error in (no error)"=w391, "local path"=w389, "remote path"=w385, "IpConf"=w392) -> ("error out"=w388:errorcluster)  [unwired: 5 in, 2 out]
          }
        }
      }
      event "Cmd_PutFile": Value Change {
        n255 = event-data() -> ("NewVal"=w393:bool)  [unwired: 1 in, 5 out]
        n256 = case shown="Faux" w393 {
          tunnel: [w396 w397] -> w394
          tunnel: w395 -> [w396 w401]
          frame False {
          }
          frame True {
            n257 = local read "Cmd_Parameters"() -> (w399:string)
            n258 = local read "WorkingDir"() -> (w400:path)
            n259 = Build Path(base path=w400, name or relative path=w399) -> (appended path=w398:path)
            n260 = local read "Tftp"() -> (w402:T1)
            n261 = call "TFTP Put File.vi"("error in (no error)"=w401, "local path"=w398, "remote path"=w399, "IpConf"=w402) -> ("error out"=w397:errorcluster)  [unwired: 5 in, 2 out]
          }
        }
      }
    }
    n262 = call "FGV_STOP.vi"("error in (no error)"=w61, "Action"=Action."GET") -> ("error out"=w62:errorcluster, "Data_OUT"=w63:bool)  [unwired: 8 in]
  }
  n263 = node-c288() -> (w6:T7)  [unwired: 4 in]
  n264 = timed-loop {
    timing: w6 -> [_]
    timing-out: [_] -> w5
    tunnel: w4 -> [w404]
    tunnel: [w407] -> w3
    stop <- w406 stop-if-true
    n265 = node-c288() -> ()  [unwired: 1 in, 1 out]
    n266 = local read "Telnet_Connected"() -> (w403:bool)
    n267 = case shown="Faux" w403 {
      tunnel: [w409 w410] -> w405
      tunnel: w404 -> [w409 w412]
      frame False {
      }
      frame True {
        n268 = local read "telnet connection"() -> (w413:T2)
        n269 = local read "Telnet_Console"() -> (w414:string)
        n270 = call "Telnet_Receive.vi"("Error In"=w412, "Console in"=w414, "telnet connection in"=w413) -> ("Error Out"=w410:errorcluster, "Console out"=w411:string)  [unwired: 4 in, 3 out]
        "Error Out" <- w410
        n271 = local write "Telnet_Console"(w411) -> ()
      }
    }
    n272 = node-c288() -> ()  [unwired: 1 in, 1 out]
    n273 = call "FGV_STOP.vi"("error in (no error)"=w405, "Action"=Action."GET") -> ("error out"=w407:errorcluster, "Data_OUT"=w406:bool)  [unwired: 8 in]
  }
  n274 = node-c288(w5) -> ()  [unwired: 1 out]
  n275 = flat-sequence {
    tunnel: w2 -> [w418]
    tunnel: [w417] -> w1
    frame #0 {
      n276 = local read "Telnet_Connected"() -> (w419:bool)
      n277 = case shown="Vrai" w419 {
        tunnel: w418 -> [w420 w423]
        tunnel: [w420 w422] -> w417
        frame False {
        }
        frame True {
          n278 = local read "telnet connection"() -> (w421:T2)
          n279 = call "Telnet_Close.vi"("Error In"=w423, "telnet connection"=w421) -> ("Error Out"=w422:errorcluster)  [unwired: 8 in, 1 out]
        }
      }
    }
  }
  n280 = Merge Errors(w1, w3) -> (w18:errorcluster)
  n281 = call <vilib>:"Clear Errors.vi"("error in (no error)"=w18) -> ("error out"=w17:errorcluster)  [unwired: 6 in]
  n282 = Destroy User Event(user event=w9, error in=w17) -> (error out=w16:errorcluster)
  n283 = Unregister For Events(event registration refnum=w8, error in=w16) -> (error out=w11:errorcluster)
  n284 = property class="App"(error in=w11) -> (error out=w14:errorcluster, "App.Kind"=w12:T3)  [unwired: 1 in, 1 out]
  n285 = Equal?(x=w12, y=T3."Run Time System" ("Application:Type")) -> (x = y?=w15:bool)
  n286 = case shown="Vrai" w15 {
    tunnel: [w424 w428] -> w10
    tunnel: w14 -> [w424 w430]
    frame False {
    }
    frame True {
      n287 = control-ref of="ce VI"() -> (w429:refnum<vi>)
      n288 = invoke class="VI" method="FA.Fermer"(reference=w429, error in=w430) -> (reference out=w426:refnum<vi>, error out=w427:errorcluster)  [unwired: 1 in, 1 out]
      n289 = Close Reference(reference=w426, error in (no error)=w427) -> (error out=w425:errorcluster)
      n290 = flat-sequence {
        tunnel: w425 -> [w433]
        tunnel: [w433] -> w428
        frame #0 {
          n291 = local read "LauncherRef"() -> (w431:refnum<vi>)
          n292 = Not A Number/Path/Refnum?(number/path/refnum=w431) -> (NaN/Path/Refnum?=w432:bool)
          n293 = case shown="Faux" w432 {
            frame False {
              n294 = Quit LabVIEW(quit? (T)=TRUE ("quitter ? (V)")) -> ()
            }
            frame True {
            }
          }
        }
      }
    }
  }
  "sortie d'erreur" <- w10
